vi "Autobalance Data Curves.vi"(10 "name or relative path":path) -> (2 "all rows":dbl[][](array[numeric]) format="%0.3f")   [LabVIEW 2009]
uses:
  <vilib>/Utility/file.llb/Read From Spreadsheet File (DBL).vi
panel:
  out "appended path":path
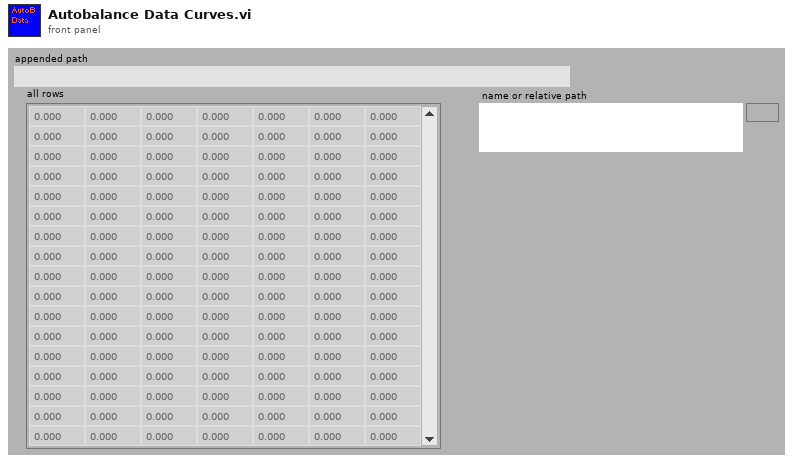
[diagram p1: front panel]
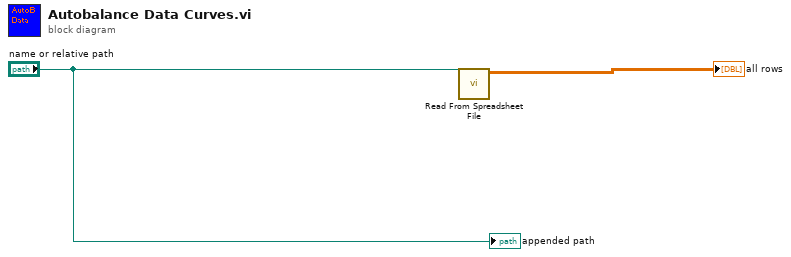
[diagram p0: block diagram]
diagram:
  n1 = call-poly <vilib>:"Read From Spreadsheet File.vi"("file path (dialog if empty)"="name or relative path") -> ("all rows"=→"all rows":dbl[][])  [unwired: 3 in, 7 out]
  "appended path" <- "name or relative path"
